vi "Module Init.vi"(8 "error in (no error)":errorcluster, 11 "DAQmxDO in":refnum<class "DAQmxDO.lvclass">) -> (0 "error out":errorcluster, 3 "DAQmxDO out":refnum<class "DAQmxDO.lvclass">)   [LabVIEW 2023, in "VolatusDAQ.lvlib" / "DAQmxDO.lvclass"]
uses:
  DAQmxDO.lvclass
  VolatusData/DataProc Options.ctl
  DAQmxDO.lvclass/DAQmxDO.ctl
  Volatus/Module/Module.lvclass/Module.ctl
  Volatus/MessageQ/MessageQ.lvclass/MessageQ.ctl
  Volatus/Module/Self Q.vi
  Volatus/MessageQ/Send.vi
  Volatus/Module/Module.lvclass
  VolatusData/Data Processor Module/Data Processor Module.lvclass
  VolatusDAQ.lvlib
  C:/dev/volatus/mts-volatus-super/libs/lv-volatus/Volatus/Module/Module.lvclass
  C:/dev/volatus/mts-volatus-super/libs/lv-volatus/VolatusDAQ/DAQmxDO/DAQmxDO.lvclass
  VolatusData/VolatusData.lvlib
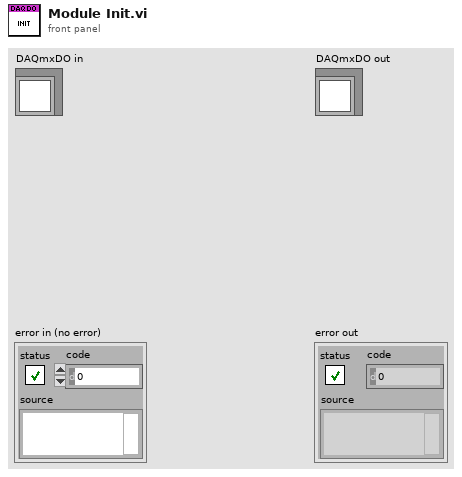
[diagram p1: front panel]
types:
  T1 = typedef "VolatusData.lvlib/DataProc Options.ctl" = cluster{"Ignore Scaling":bool}
  T2 = typedef "VolatusDAQConfig.lvlib/Sampling Config.ctl" = cluster{"Rate":dbl, "Chunk Size":i32}
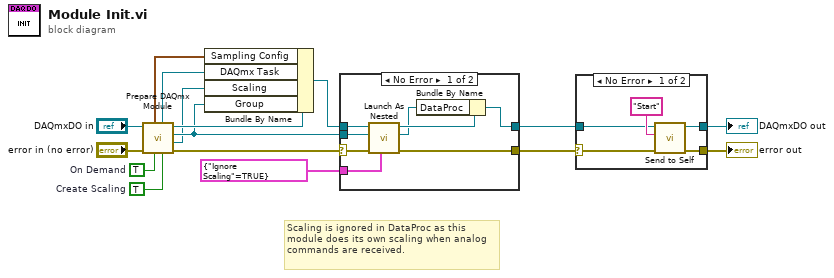
[diagram p0: block diagram]
diagram:
  w6 = TRUE  # On Demand
  w7 = TRUE  # Create Scaling
  # "Scaling is ignored in DataProc as this module does its own scaling when analog commands are received."
  n1 = call "Prepare DAQmx Module.vi"("Create Scaling (F)"=w7, "On Demand (F)"=w6, "error in (no error)"="error in (no error)", "Module in"="DAQmxDO in") -> ("error out"=w13:errorcluster, "Scaling"=w10:refnum<class "Scaling.lvclass">, "Group"=w11:refnum<class "Group DBL.lvclass">, "Module out"=w16:refnum<class "DAQmxDO.lvclass">, "DAQmx Task"=w15:refnum<k21>, "Sampling Config"=w14:T2)  [unwired: 2 in]
  n2 = Bundle By Name(cluster=w16, "Sampling Config"=w14, "DAQmx Task"=w15, "Scaling"=w10, "Group"=w11) -> (w12:refnum<class "DAQmxDO.lvclass">)
  n3 = case shown="No Error" w13 {
    selector: w13 -> [w24 w25]
    tunnel: w12 -> [w23 w26]
    tunnel: w11 -> [w22 _]
    tunnel: [w21 w25] -> w8
    tunnel: [w18 w26] -> w9
    tunnel: T1 {"Ignore Scaling"=TRUE} ("DataProc Options") -> [w17 _]
    frame No Error {
      n4 = call "Launch As Nested.vi"("DataProc Options"=w17, "error in (no error)"=w24, "Group"=w22, "Parent in"=w23) -> ("error out"=w21:errorcluster, "MessageQ"=w19:refnum<class "MessageQ.lvclass">, "Parent out"=w20:refnum<class "DAQmxDO.lvclass">)  [unwired: 5 in]
      n5 = Bundle By Name(cluster=w20, "DataProc"=w19) -> (w18:refnum<class "DAQmxDO.lvclass">)
    }
    frame Error {
    }
  }
  n6 = case shown="No Error" w8 {
    selector: w8 -> [w27 w33]
    tunnel: [w31 w33] -> w2
    tunnel: w9 -> [w28 w32]
    tunnel: [w30 w32] -> w3
    frame No Error {
      n7 = call "Send to Self.vi"("error in (no error)"=w27, "Message ID"="Start", "Module in"=w28) -> ("error out"=w31:errorcluster, "Module out"=w30:refnum<class "DAQmxDO.lvclass">)  [unwired: 7 in]
    }
    frame Error {
    }
  }
  "error out" <- w2
  "DAQmxDO out" <- w3
